vi "rotation.vi"(8 "error in (no error)":errorcluster, 11 "Angle":dbl) -> (0 "error out":errorcluster)   [LabVIEW 2016]
uses:
  <vilib>/myRIO/Common/Instrument Driver Framework/myRIO v1.0/Encoder/typedefs/Encoder Signal Mode.ctl
  <vilib>/myRIO/Instrument Drivers/Onboard IO/Encoder/typedefs/Encoder Reference.ctl
  <vilib>/myRIO/Common/Instrument Driver Framework/Utilities/typedefs/myRIO Generic Hardware Reference.ctl
  <vilib>/myRIO/Common/Instrument Driver Framework/Utilities/typedefs/Hardware Version Enum.ctl
  <vilib>/myRIO/Common/Instrument Driver Framework/Utilities/typedefs/myRIO v1.0 Reference.ctl
  <vilib>/myRIO/Common/Instrument Driver Framework/Utilities/typedefs/Generic FPGA Reference.ctl
  <vilib>/myRIO/Common/Instrument Driver Framework/myRIO v1.0/Encoder/typedefs/Encoder Channels Enum.ctl
  <vilib>/myRIO/Common/Instrument Driver Framework/myRIO v1.0/Encoder/typedefs/Encoder Configuration v1.0.ctl
  <vilib>/userdefined/High Color/nirio_resource_hc.ctl
  <vilib>/myRIO/Instrument Drivers/Onboard IO/PWM/typedefs/PWM Reference.ctl
  <vilib>/myRIO/Common/Instrument Driver Framework/myRIO v1.0/PWM/typedefs/PWM Channels Enum.ctl
  <vilib>/myRIO/Instrument Drivers/Onboard IO/PWM/typedefs/PWM Configuration.ctl
  <vilib>/myRIO/Instrument Drivers/Onboard IO/DIO/typedefs/DIO Reference.ctl
  <vilib>/myRIO/Common/Instrument Driver Framework/myRIO v1.0/DIO/typedefs/DIO Channels List.ctl
  <vilib>/myRIO/Common/Instrument Driver Framework/myRIO v1.0/DIO/typedefs/DIO Channels Enum.ctl
  <vilib>/myRIO/Common/Instrument Driver Framework/Utilities/vis/Is FPGA Ref Available.vi
  <vilib>/myRIO/Common/Instrument Driver Framework/myRIO v1.0/Encoder/vis/myRIO v1.1 Open Encoder.vi
  <vilib>/myRIO/Instrument Drivers/Onboard IO/Encoder/vis/Read.vi
  <vilib>/myRIO/Common/Instrument Driver Framework/myRIO v1.0/PWM/vis/myRIO v1.1 Open PWM.vi
  <vilib>/myRIO/Instrument Drivers/Onboard IO/PWM/vis/Set Duty Cycle and Frequency.vi
  <vilib>/myRIO/Common/Instrument Driver Framework/myRIO v1.0/DIO/vis/myRIO v1.1 Open DIO.vi
  <vilib>/myRIO/Instrument Drivers/Onboard IO/DIO/vis/Write.vi
  <vilib>/myRIO/Common/Instrument Driver Framework/Utilities/vis/Validate Channels.vi
  <vilib>/myRIO/Common/Instrument Driver Framework/myRIO v1.0/Encoder/vis/myRIO v1.0 Reserve Encoder.vi
  <vilib>/myRIO/Common/Instrument Driver Framework/myRIO v1.0/PWM/vis/myRIO v1.0 Reserve PWM.vi
  <vilib>/myRIO/Common/Instrument Driver Framework/myRIO v1.0/DIO/vis/myRIO v1.0 Reserve DIO.vi
  <vilib>/myRIO/Common/Instrument Driver Framework/myRIO v1.0/Encoder/vis/myRIO v1.0 Build MUX Configuration Encoder.vi
  <vilib>/myRIO/Common/Instrument Driver Framework/myRIO v1.0/Resource Manager/vis/myRIO v1.0 Reserve Channel List.vi
  <vilib>/myRIO/Common/Instrument Driver Framework/myRIO v1.0/PWM/vis/myRIO v1.0 Build MUX Configuration PWM.vi
  <vilib>/myRIO/Common/Instrument Driver Framework/myRIO v1.0/DIO/vis/myRIO v1.0 Build MUX Configuration DIO.vi
  <vilib>/myRIO/Common/Instrument Driver Framework/myRIO v1.0/Resource Manager/vis/myRIO v1.0 Create Configuration List.vi
  <vilib>/myRIO/Common/Instrument Driver Framework/myRIO v1.0/Resource Manager/vis/myRIO v1.0 Reserve Channel.vi
  <vilib>/myRIO/Common/Instrument Driver Framework/myRIO v1.0/Resource Manager/vis/myRIO v1.0 Unreserve Channel.vi
  <vilib>/myRIO/Common/Instrument Driver Framework/myRIO v1.0/Resource Manager/vis/myRIO v1.0 Build Mutex Name.vi
  <vilib>/Utility/VariantDataType/GetNumericInfo.vi
  <vilib>/Utility/error.llb/Error Cluster From Error Code.vi
  <vilib>/myRIO/Common/Instrument Driver Framework/myRIO v1.0/myRIO v1.1 Open.vi
  <vilib>/myRIO/Common/Instrument Driver Framework/Utilities/vis/IO Manager.vi
  <vilib>/myRIO/Common/Instrument Driver Framework/Utilities/vis/Configuration Manager.vi
  <vilib>/myRIO/Common/Instrument Driver Framework/myRIO v1.0/Resource Manager/vis/myRIO v1.0 Configure IO.vi
  <vilib>/myRIO/Common/Instrument Driver Framework/myRIO v1.0/myRIO v1.0 Close.vi
  <vilib>/myRIO/Common/Instrument Driver Framework/myRIO v1.0/Encoder/vis/myRIO v1.0 Configure Encoder.vi
  <vilib>/myRIO/Common/Instrument Driver Framework/myRIO v1.0/Encoder/vis/myRIO v1.0 Read Encoder.vi
  <vilib>/imath/engines/lvmath2/RunTimeEngine/BuiltInFunctions/abs/NIMS_abs(signed).vi
  <instcachedir>/0/NIMS_abs(signed)_C4FCB8E6058B49B797C7C8D53CA5F6EC.lvgen/NIMS_abs(signed)_C4FCB8E6058B49B797C7C8D53CA5F6EC_007.vi
  <vilib>/imath/engines/lvmath2/RunTimeEngine/NodeEndStatement/NIMS_NodeEndStatement_Output.vi
  <instcachedir>/0/NIMS_NodeEndStatement_Output_53EC0D466D134D7ABD903AC30B43404B.lvgen/NIMS_NodeEndStatement_Output_53EC0D466D134D7ABD903AC30B43404B_001.vi
  <vilib>/imath/engines/lvmath2/RunTimeEngine/ErrorHandling/NIMS_Finalize Error.vi
  <vilib>/myRIO/Common/Instrument Driver Framework/myRIO v1.0/PWM/vis/myRIO v1.0 Write PWM.vi
  <vilib>/myRIO/Common/Instrument Driver Framework/myRIO v1.0/DIO/vis/myRIO v1.0 Write DIO.vi
  <vilib>/myRIO/Express VI/Onboard IO/Encoder/Encoder Express VI.xnode
  <vilib>/myRIO/Instrument Drivers/Onboard IO/Encoder/vis/myRIO Encoder Open.xnode
  <vilib>/myRIO/Common/Instrument Driver Framework/myRIO v1.0/Encoder/typedefs/Encoder Count Direction Enum.ctl
  <vilib>/myRIO/Express VI/Onboard IO/PWM/PWM Express VI.xnode
  <vilib>/myRIO/Instrument Drivers/Onboard IO/PWM/vis/myRIO PWM Open.xnode
  <vilib>/myRIO/Express VI/Onboard IO/DO/DO Express VI.xnode
  <vilib>/myRIO/Instrument Drivers/Onboard IO/DIO/vis/myRIO DIO Open.xnode
  <vilib>/myRIO/Instrument Drivers/Onboard IO/PWM/PWM.lvlib
  <vilib>/myRIO/Instrument Drivers/Onboard IO/Encoder/Encoder.lvlib
  <vilib>/myRIO/Instrument Drivers/Onboard IO/DIO/DIO.lvlib
panel:
  in  "[ESC]":bool
  in  "PWM  [%]":dbl(slide)=25.0 scale=-100.0..100.0
  out "Counter Right":i32
  out "Need":dbl
  out "PWM Right":dbl
  out "PWM Left":dbl
  out "Counter Left":i32
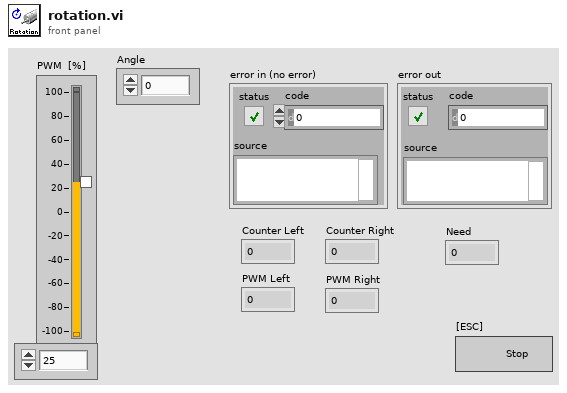
[diagram p1: front panel]
types:
  T1 = typedef "Encoder.lvlib/Encoder Reference.ctl" = cluster{"myRIO Reference":T2, "Encoder Channels Enum":T6}
  T2 = typedef "myRIO Generic Hardware Reference.ctl" = cluster{"myRIO Model":T3, "myRIO Hardware Reference":T4}
  T3 = typedef "Hardware Version Enum.ctl" = enum16{"Unknown", "myRIO-1900", "myRIO-1950", "roboRIO", "NI ELVIS RIO CM"}
  T4 = typedef "myRIO v1.0 Reference.ctl" = cluster{"Generic FPGA Reference":T5, "Allow multiple opens":bool}
  T5 = typedef "Generic FPGA Reference.ctl" = refnum<k20>
  T6 = typedef "Encoder Channels Enum.ctl" = enum16{"Not Connected", "C/ENC0", "C/ENC1", "A/ENC", "B/ENC", "DIO/ENC0", "DIO/ENC1", "DIO/ENC2", "DIO/ENC3", "DIO/ENC4"}
  T7 = typedef "Encoder Signal Mode.ctl" = enum16{"Quadrature phase signal", "Step and direction signal"}
  T8 = typedef "nirio_resource_hc.ctl" = tag
  T9 = typedef "DIO.lvlib/DIO Reference.ctl" = cluster{"myRIO Reference":T2, "DIO Channels List":T10}
  T10 = typedef "DIO Channels List.ctl" = T11[]
  T11 = typedef "DIO Channels Enum.ctl" = enum16{"Not Connected", "C/DIO0", "C/DIO1", "C/DIO2", "C/DIO3", "C/DIO4", "C/DIO5", "C/DIO6", "C/DIO7", "A/DIO0", "A/DIO1", "A/DIO2", "A/DIO3", "A/DIO4", "A/DIO5", "A/DIO6", "A/DIO7", "A/DIO8", "A/DIO9", "A/DIO10", "A/DIO11", "A/DIO12", "A/DIO13", "A/DIO14", "A/DIO15", "B/DIO0", "B/DIO1", "B/DIO2", "B/DIO3", "B/DIO4", "B/DIO5", "B/DIO6", "B/DIO7", "B/DIO8", "B/DIO9", "B/DIO10", "B/DIO11", "B/DIO12", "B/DIO13", "B/DIO14", "B/DIO15", "LED0", "LED1", "LED2", "LED3", "Button0", "DIO/DIO0", "DIO/DIO1", "DIO/DIO2", "DIO/DIO3", "DIO/DIO4", "DIO/DIO5", "DIO/DIO6", "DIO/DIO7", "DIO/DIO8", "DIO/DIO9", "SPI/CS0", "SPI/CS1", "SPI/CS2", "SPI/CS3", "LED RADIO (Green)", "LED RADIO (Red)", "LED COMM (Green)", "LED COMM (Red)", "LED MODE (Green)", "LED MODE (Red)"}
  T12 = typedef "PWM.lvlib/PWM Reference.ctl" = cluster{"myRIO Reference":T2, "PWM Channels Enum":T13, "PWM Configuration":T14}
  T13 = typedef "PWM Channels Enum.ctl" = enum16{"Not Connected", "C/PWM0", "C/PWM1", "A/PWM0", "A/PWM1", "A/PWM2", "B/PWM0", "B/PWM1", "B/PWM2", "PWM/PWM0", "PWM/PWM1", "PWM/PWM2", "PWM/PWM3", "PWM/PWM4", "PWM/PWM5", "PWM/PWM6", "PWM/PWM7", "PWM/PWM8", "PWM/PWM9"}
  T14 = typedef "PWM.lvlib/PWM Configuration.ctl" = cluster{"Frequency":dbl, "Duty Cycle":dbl}
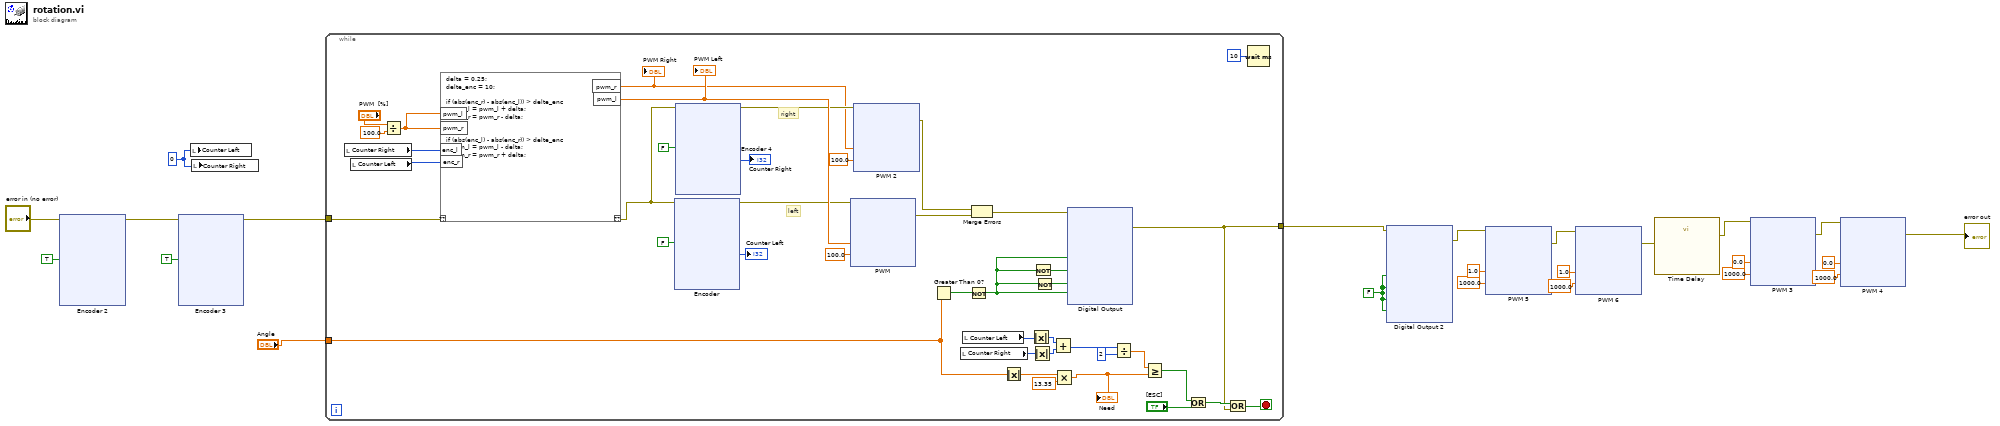
[diagram p0: block diagram]
diagram:
  w11 = FALSE
  w18 = 0
  n1 = xnode "Encoder 2"("Reset Counter"=TRUE, "error in (no error)"="error in (no error)") -> ("error out"=w20:errorcluster)  [unwired: 3 out]
  n2 = xnode "Encoder 3"("Reset Counter"=TRUE, "error in (no error)"=w20) -> ("error out"=w19:errorcluster)  [unwired: 3 out]
  n3 = local write "Counter Left"(w18) -> ()
  n4 = local write "Counter Right"(w18) -> ()
  n5 = while {
    tunnel: w19 -> [w59]
    tunnel: "Angle" -> [w40]
    tunnel: [w51] -> w10
    stop <- w32 stop-if-true
    # "left"
    # "right"
    n6 = local read "Counter Right"() -> (w49:i32)
    n7 = local read "Counter Left"() -> (w43:i32)
    n8 = Divide(x="PWM  [%]", y=100.0) -> (x/y=w60:dbl)
    n9 = mathscript code="delta = 0.25;\ndelte_enc = 10;\n\nif (abs(enc_r) - abs(enc_l)) > delte_enc\n  pwm_l = pwm_l + delta;\n  pwm_r = pwm_r - delta;\nend\n\nif (abs(enc_l) - abs(enc_r)) > delte_enc\n  pwm_l = pwm_l - delta;\n  pwm_r = pwm_r + delta;\nend"("??"=w59, "pwm_l"=w60, "pwm_r"=w60, "enc_l"=w49, "enc_r"=w43) -> ("??"=w47:errorcluster, "pwm_l"=w55:dbl, "pwm_r"=w28:dbl)
    "PWM Right" <- w28
    "PWM Left" <- w55
    n10 = xnode "Encoder"("Reset Counter"=FALSE, "error in (no error)"=w47) -> ("Counter Value"=→"Counter Left":i32, "error out"=w46:errorcluster)  [unwired: 2 out]
    n11 = xnode "Encoder 4"("Reset Counter"=FALSE, "error in (no error)"=w47) -> ("Counter Value"=→"Counter Right":i32, "error out"=w45:errorcluster)  [unwired: 2 out]
    n12 = xnode "PWM"("Duty Cycle"=w55, "Frequency [Hz]"=100.0, "error in (no error)"=w46) -> ("error out"=w57:errorcluster)
    n13 = xnode "PWM 2"("Duty Cycle"=w28, "Frequency [Hz]"=100.0, "error in (no error)"=w45) -> ("error out"=w58:errorcluster)
    n14 = Greater Than 0?(x=w40) -> (x > 0?=w50:bool)
    n15 = local read "Counter Right"() -> (w38:i32)
    n16 = local read "Counter Left"() -> (w39:i32)
    n17 = Not(x=w50) -> (.not. x?=w24:bool)
    n18 = Merge Errors(w58, w57) -> (w56:errorcluster)
    n19 = Absolute Value(x=w40) -> (abs(x)=w33:dbl)
    n20 = Absolute Value(x=w39) -> (abs(x)=w36:i32)
    n21 = Absolute Value(x=w38) -> (abs(x)=w37:i32)
    n22 = Not(x=w24) -> (.not. x?=w31:bool)
    n23 = Not(x=w24) -> (.not. x?=w25:bool)
    n24 = Add(x=w36, y=w37) -> (x+y=w35:i32)
    n25 = Multiply(x=w33, y=13.35) -> (x*y=w30:dbl)
    "Need" <- w30
    n26 = xnode "Digital Output"("M0 Enable (A/DIO5 (Pin 21))"=w24, "M0 Reverse (A/DIO6 (Pin 23))"=w31, "M1 Enable (A/DIO7 (Pin 25))"=w25, "M1 Reverse (A/DIO13 (Pin 26))"=w24, "error in (no error)"=w56) -> ("error out"=w51:errorcluster)
    n27 = Divide(x=w35, y=2) -> (x/y=w29:dbl)
    n28 = Greater Or Equal?(x=w29, y=w30) -> (x >= y?=w42:bool)
    n29 = Or(x=w42, y="[ESC]") -> (x .or. y?=w61:bool)
    n30 = Or(x=w61, y=w51) -> (x .or. y?=w32:bool)
    n31 = Wait (ms)(milliseconds to wait=u32 10) -> ()  [unwired: 1 out]
  }
  n32 = xnode "Digital Output 2"("M0 Enable (A/DIO5 (Pin 21))"=w11, "M0 Reverse (A/DIO6 (Pin 23))"=w11, "M1 Enable (A/DIO7 (Pin 25))"=w11, "M1 Reverse (A/DIO13 (Pin 26))"=w11, "error in (no error)"=w10) -> ("error out"=w5:errorcluster)
  n33 = xnode "PWM 5"("Duty Cycle"=1.0, "Frequency [Hz]"=1000.0, "error in (no error)"=w5) -> ("error out"=w4:errorcluster)
  n34 = xnode "PWM 6"("Duty Cycle"=1.0, "Frequency [Hz]"=1000.0, "error in (no error)"=w4) -> ("error out"=w3:errorcluster)
  n35 = call "Time Delay"("error in (no error)"=w3) -> ("error out"=w13:errorcluster)  [unwired: 10 in]
  n36 = xnode "PWM 3"("Duty Cycle"=0.0, "Frequency [Hz]"=1000.0, "error in (no error)"=w13) -> ("error out"=w12:errorcluster)
  n37 = xnode "PWM 4"("Duty Cycle"=0.0, "Frequency [Hz]"=1000.0, "error in (no error)"=w12) -> ("error out"=→"error out":errorcluster)
